vi "Compile APU.vi"(8 "error in (no error)":errorcluster, 10 "Channel Descriptors in":T1, 11 "Custom Device Ref in":T8 format="%.0x") -> (0 "error out":errorcluster, 1 "IncrementRate":i64, 2 "Channel Descriptors out":T1, 3 "Custom Device Ref out":T8 format="%.0x")   [LabVIEW 2011, in "Engine Sim System Explorer.lvlib"]
uses:
  Engine Sim System Explorer.lvlib
  <vilib>/NI Veristand/Custom Device API/Custom Device Item Ref.ctl
  Shared/Channel Descriptors.ctl
  Shared/FPGA Write Descriptor.ctl
  Shared/InputChannelTypes.ctl
  <vilib>/rvi/DataTransferAndStorage/Container/Common/niFpgaDataTypeControl.ctl
  Shared/FPGA Read Descriptor.ctl
  Shared/OutputChannelTypes.ctl
  Shared/Status Chan Descriptor.ctl
  <vilib>/NI Veristand/Custom Device Tools/Custom Device Utility Library/NI VeriStand - Search for Item by Name.vi
  Shared/Engine Simulation Global.vi
  <vilib>/NI Veristand/Custom Device API/Get Item Property (Double).vi
  <vilib>/NI Veristand/Custom Device API/Custom Device API.lvlib
  Engine Simulation Shared.lvlib
  <userlib>/AES/RT/AES RT.lvlib
  <vilib>/NI Veristand/Custom Device Tools/Custom Device Utility Library/Custom Device Utility Library.lvlib
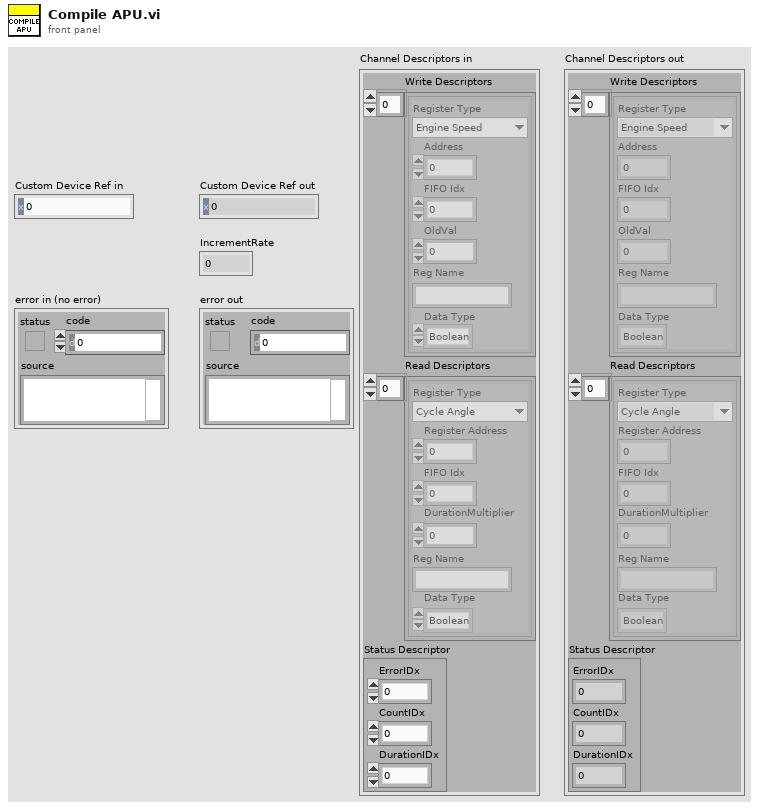
[diagram p1: front panel]
types:
  T1 = typedef "Engine Simulation Shared.lvlib/Channel Descriptors.ctl" = cluster{"Write Descriptors":T2[], "Read Descriptors":T5[], "Status Descriptor":T7}
  T2 = typedef "Engine Simulation Shared.lvlib/FPGA Write Descriptor.ctl" = cluster{"Register Type":T3, "Address":u32, "FIFO Idx":i32, "OldVal":dbl, "Reg Name":string, "Data Type":T4}
  T3 = typedef "Engine Simulation Shared.lvlib/InputChannelTypes.ctl" = enum16{"Engine Speed", "Offset"}
  T4 = typedef "niFpgaDataTypeControl.ctl" = enum32{"Boolean", "I8", "I16", "I32", "I64", "U8", "U16", "U32", "U64", "FXP", "CustomControl"}
  T5 = typedef "Engine Simulation Shared.lvlib/FPGA Read Descriptor.ctl" = cluster{"Register Type":T6, "Register Address":u32, "FIFO Idx":i32, "DurationMultiplier":dbl, "Reg Name":string, "Data Type":T4}
  T6 = typedef "Engine Simulation Shared.lvlib/OutputChannelTypes.ctl" = enum16{"Cycle Angle", "Crank Angle", "Time Duration", "Angle Duration", "Start Angle", "End Angle"}
  T7 = typedef "Engine Simulation Shared.lvlib/Status Chan Descriptor.ctl" = cluster{"ErrorIDx":i32, "CountIDx":i32, "DurationIDx":i32}
  T8 = typedef "Custom Device API.lvlib/Custom Device Item Ref.ctl" = u64
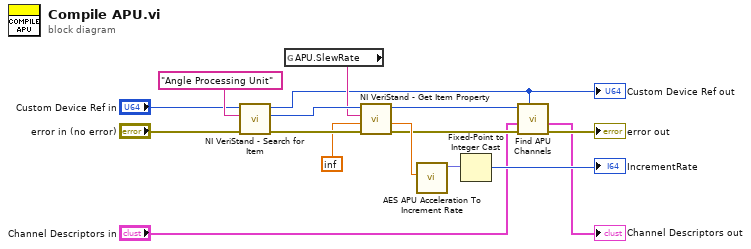
[diagram p0: block diagram]
diagram:
  n1 = call-poly <vilib>:"NI VeriStand - Search for Item.vi"("error in"="error in (no error)", "Item Name"="Angle Processing Unit", "Section Ref in"="Custom Device Ref in") -> ("error out"=w16:errorcluster, "Item Ref"=w15:T8, "Section Ref out"=w4:T8)  [unwired: 5 in, 1 out]
  "Custom Device Ref out" <- w4
  n2 = global read "Engine Simulation Global.vi" "APU.SlewRate"() -> (w7:string)
  n3 = call-poly <vilib>:"NI VeriStand - Get Item Property.vi"("error in (no error)"=w16, "Default Value"=inf, "Property Name"=w7, "Item Ref in"=w15) -> ("error out"=w6:errorcluster, "Value"=w9:dbl, "Item Ref out"=w3:T8)  [unwired: 4 in, 1 out]
  n4 = call <userlib>:"AES APU Acceleration To Increment Rate.vi"("acceleration (RPM/sec)"=w9) -> ("increment rate"=w10:fxp<+/-,47,-4>)  [unwired: 10 in]
  n5 = Fixed-Point to Integer Cast(1:w10) -> (0:→"IncrementRate":i64)
  n6 = call "Find APU Channels.vi"("Custom Device Ref"=w4, "error in (no error)"=w6, "Channel Descriptors in"="Channel Descriptors in", "APU ref"=w3) -> ("error out"=→"error out":errorcluster, "Channel Descriptors out"=→"Channel Descriptors out":T1)  [unwired: 6 in]
